vi "Picture_Clean_Data_Array.vi"(8 "Input Cluster":T6, 11 "Boolean":bool) -> (0 "output cluster":T6)   [LabVIEW 2009]
uses:
  atmcd32d.llb/AcquisitionMode_mode typedef.ctl
  atmcd32d.llb/ReadMode_mode typedef.ctl
  atmcd32d.llb/TriggerMode_mode typedef.ctl
  atmcd32d.llb/Shutter_type typedef.ctl
  atmcd32d.llb/Shutter_mode typedef.ctl
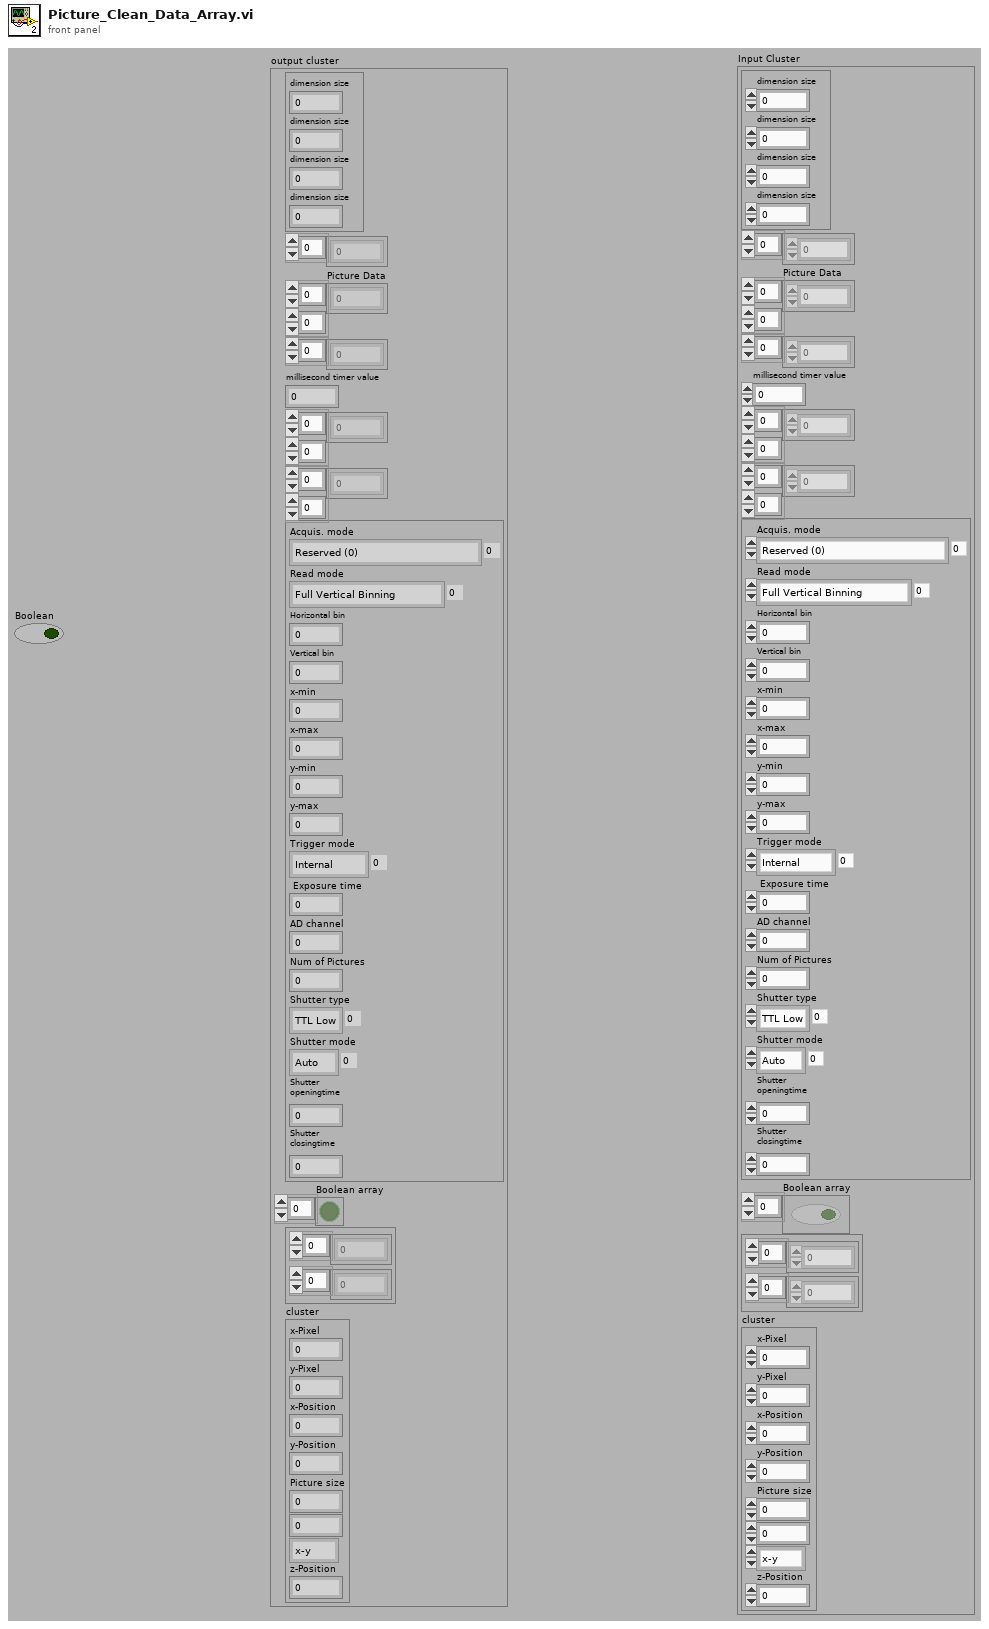
[diagram p1: front panel]
types:
  T1 = typedef "AcquisitionMode_mode typedef.ctl" = enum16{"Reserved (0)", "Single Scan", "Accumulate", "Kinetics", "Fast Kinetics", "Run Till Abort", "Reserved (6)", "Reserved (7)", "Reserved (8)", "Time Delayed Integration"}
  T2 = typedef "ReadMode_mode typedef.ctl" = enum16{"Full Vertical Binning", "Multi-Track", "Random-Track", "Single-Track", "Image"}
  T3 = typedef "TriggerMode_mode typedef.ctl" = enum16{"Internal", "External", "N/A (2)", "N/A (3)", "N/A (4)", "N/A (5)", "External Start"}
  T4 = typedef "Shutter_type typedef.ctl" = enum16{"TTL Low", "TTL High"}
  T5 = typedef "Shutter_mode typedef.ctl" = enum16{"Auto", "Open", "Close"}
  T6 = cluster{cluster{"dimension size":i32, "dimension size":i32, "dimension size":i32, "dimension size":i32}, i32[], "Picture Data":dbl[][], u32[], "millisecond timer value":u32, dbl[][], i32[][], cluster{"Acquis. mode":T1, "Read mode":T2, "Horizontal bin":i32, "Vertical bin":i32, "x-min":i32, "x-max":i32, "y-min":i32, "y-max":i32, "Trigger mode":T3, " Exposure time":sgl, "AD channel":i32, "Num of Pictures":i32, "Shutter type":T4, "Shutter mode":T5, "Shutter\nopeningtime":i32, "Shutter\nclosingtime":i32}, "Boolean array":bool[], cluster{dbl[], dbl[]}, "cluster":cluster{"x-Pixel":u16, "y-Pixel":u16, "x-Position":dbl, "y-Position":dbl, "Picture size":dbl, dbl, enum32{"x-y", "x-z", "y-z"}, "z-Position":dbl}}
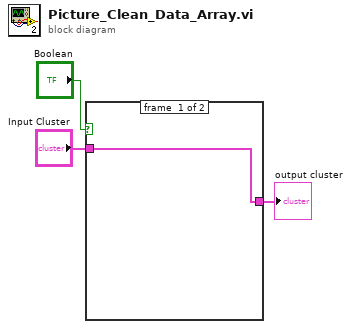
[diagram p0: block diagram]
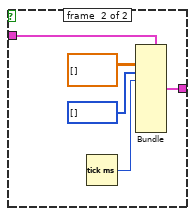
[diagram p2: hidden frame]
diagram:
  n1 = case shown="True" "Boolean" {
    tunnel: "Input Cluster" -> [w4 w5]
    tunnel: [w4 w8] -> w1
    frame #0 {
    }
    frame #1 {
      n2 = Tick Count (ms)() -> (millisecond timer value=w6:u32)
      n3 = Bundle(cluster=w5, "Picture Data"=dbl[][] [], u32[] [], "millisecond timer value"=w6) -> (w8:T6)  [unwired: 8 out]
    }
  }
  "output cluster" <- w1
